vi "AlliGator Get Square Gated IRF Analysis Cursors.vi"(8 "Error In":errorcluster, 11 "XYGraph in":refnum<vi>) -> (0 "Error Out":errorcluster, 1 "5 Cursors available?":bool, 2 "Cursor Names Array":string[](array[string]), 3 "Cursor Positions Array":dbl[](array[numeric]))   [LabVIEW 2021, in "AlliGator Decay Analysis.lvlib" / "AlliGator IRF.lvlib"]
doc: "Gets locations and names of the 5 cursors needed to define the regions of a square gate fit."
uses:
  AlliGator IRF.lvlib
panel:
  out "Message":string="Operation stopped because:\nAt least 4 cursors with names tr1, tr2, tf1 and tf2 need to be defined in the Fluorescence Decay Graph."
  # "see the AlliGator License on the block diagram (Ctrl+E or Window:Show Block Diagram)"
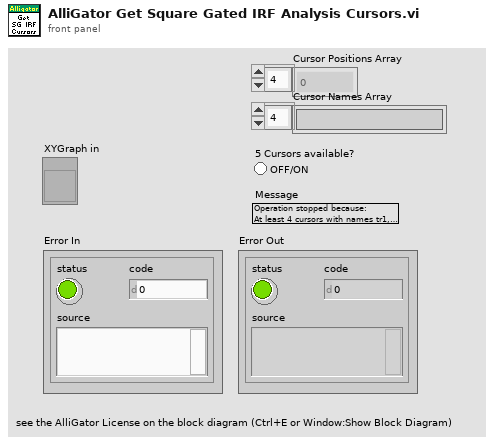
[diagram p1: front panel]
types:
  T1 = typedef "LVCursorListTypeDef.ctl" = cluster{"Name":string, "Color":u32, "Style":u8, "Point Style":u8, "Name Visible":bool, "Allow Drag":bool, "Cursor Mode":u32, "Plot":i32, "Index":i32, "Position":cluster{"X":dbl, "Y":dbl}, "X Scale":u32, "Y Scale":u32, "Watch Plots":i32[], "Watch All Plots":bool, "Plot Area":i32, "Label Offset":cluster{"X":dbl, "Y":dbl}}[]
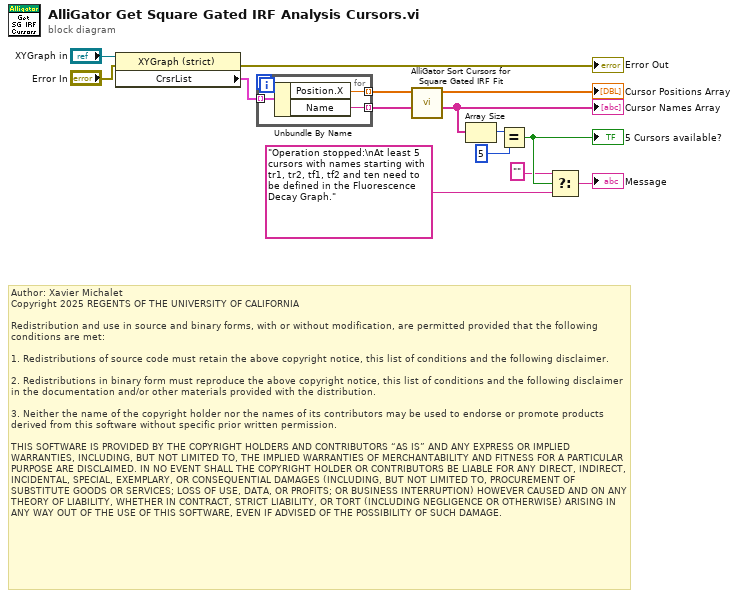
[diagram p0: block diagram]
diagram:
  # "Author: Xavier Michalet\nCopyright 2025 REGENTS OF THE UNIVERSITY OF CALIFORNIA\n\nRedistribution and use in source and binary forms, with or without modification, are permitted provided that the following conditions are met:\n\n1. Redistributions of source code must retain the above copyright notice, this list of conditions and the following disclaimer.\n\n2. Redistributions in binary form must reproduce the above copyright notice, this list of conditions and the following disclaimer in the documentation and/or other materials provided with the distribution.\n\n3. Neither the name of the copyright holder nor the names of its contributors may be used to endorse or promote products derived from this software without specific prior written permission.\n\nTHIS SOFTWARE IS PROVIDED BY THE COPYRIGHT HOLDERS AND CONTRIBUTORS “AS IS” AND ANY EXPRESS OR IMPLIED WARRANTIES, INCLUDING, BUT NOT LIMITED TO, THE IMPLIED WARRANTIES OF MERCHANTABILITY AND FITNESS FOR A PARTICULAR PURPOSE ARE DISCLAIMED. IN NO EVENT SHALL THE COPYRIGHT HOLDER OR CONTRIBUTORS BE LIABLE FOR ANY DIRECT, INDIRECT, INCIDENTAL, SPECIAL, EXEMPLARY, OR CONSEQUENTIAL DAMAGES (INCLUDING, BUT NOT LIMITED TO, PROCUREMENT OF SUBSTITUTE GOODS OR SERVICES; LOSS OF USE, DATA, OR PROFITS; OR BUSINESS INTERRUPTION) HOWEVER CAUSED AND ON ANY THEORY OF LIABILITY, WHETHER IN CONTRACT, STRICT LIABILITY, OR TORT (INCLUDING NEGLIGENCE OR OTHERWISE) ARISING IN ANY WAY OUT OF THE USE OF THIS SOFTWARE, EVEN IF ADVISED OF THE POSSIBILITY OF SUCH DAMAGE."
  n1 = property class="XYGraph (strict)"(reference="XYGraph in", error in="Error In") -> (error out=→"Error Out":errorcluster, "CrsrList"=w4:T1)  [unwired: 1 out]
  n2 = for {
    tunnel: w4 -> [w17] mode=indexing
    tunnel: [w16] -> w2 mode=indexing
    tunnel: [w15] -> w1 mode=indexing
    n3 = Unbundle By Name(w17) -> ("Position.X"=w16:dbl, "Name"=w15:string)
  }
  n4 = call "AlliGator Sort Cursors for Square Gated IRF Fit.vi"("Cursor Name Array in"=w1, "Cursor Position Array in"=w2) -> ("Sorted Cursor Name Array"=w3:string[], "Sorted Cursor Position Array"=→"Cursor Positions Array":dbl[])  [unwired: 8 in]
  "Cursor Names Array" <- w3
  n5 = Array Size(array=w3) -> (size(s)=w12:i32)
  n6 = Equal?(x=w12, y=5) -> (x = y?=w11:bool)
  "5 Cursors available?" <- w11
  n7 = Select(t="", s=w11, f="Operation stopped:\nAt least 5 cursors with names starting with tr1, tr2, tf1, tf2 and ten need to be defined in the Fluorescence Decay Graph.") -> (s? t:f=→"Message":string)
